vi "Led Control.vi"   [LabVIEW 2013]
uses:
  <vilib>/Rock Robotics/WPI/DriverStation/WPI_DriverStationAllianceInfo.ctl
  <vilib>/Rock Robotics/WPI/Relay/WPI_RelayValue.ctl
types:
  T1 = typedef "WPI_DriverStationAllianceInfo.ctl" = enum16{"Red", "Blue", "Invalid"}
  T2 = typedef "WPI_RelayValue.ctl" = enum16{"Off", "On", "Forward", "Reverse"}
  T3 = typedef "WPI_RelayDevRef.ctl" = cluster{"DevStatus":errorcluster, "Relay Channel":T4, "Digital Module":T5, "Relay Direction":T6}
  T4 = typedef "FPGA_DIORelayChannel.ctl" = enum8{"Relay 1", "Relay 2", "Relay 3", "Relay 4", "Relay 5", "Relay 6", "Relay 7", "Relay 8", "Invalid"}
  T5 = typedef "FPGA_TypedefDigitalModule.ctl" = enum16{"Digital Module 1", "Digital Module 2"}
  T6 = typedef "WPI_RelayDirection.ctl" = enum16{"Both directions", "Forward only", "Reverse only"}
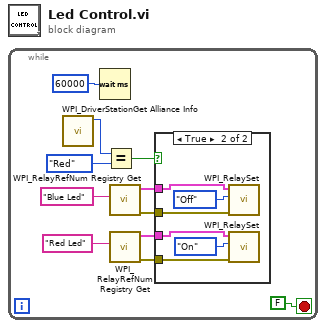
[diagram p0: block diagram]
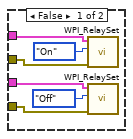
[diagram p2: hidden frame]
diagram:
  n1 = while {
    stop <- FALSE stop-if-true
    n2 = call <vilib>:"WPI_DriverStationGet Alliance Info.vi"() -> ("Alliance"=w6:T1)  [unwired: 10 in, 1 out]
    n3 = Wait (ms)(milliseconds to wait=u32 60000) -> ()  [unwired: 1 out]
    n4 = Equal?(x=w6, y=WPI_DriverStationAllianceInfo."Red" ("Alliance")) -> (x = y?=w7:bool)
    n5 = call <vilib>:"WPI_RelayRefNum Registry Get.vi"("refnum name"="Blue Led") -> ("error out"=w1:errorcluster, "RelayDevRef"=w2:T3)  [unwired: 9 in]
    n6 = call <vilib>:"WPI_RelayRefNum Registry Get.vi"("refnum name"="Red Led") -> ("error out"=w3:errorcluster, "RelayDevRef"=w4:T3)  [unwired: 9 in]
    n7 = case shown="True" w7 {
      tunnel: w4 -> [w13 w23]
      tunnel: w3 -> [w12 w22]
      tunnel: w2 -> [w15 w19]
      tunnel: w1 -> [w14 w18]
      frame False {
        n8 = call <vilib>:"WPI_RelaySet.vi"("error in (no error)"=w14, "RelayValue"=WPI_RelayValue."On", "RelayDevRef"=w15) -> ()  [unwired: 7 in, 2 out]
        n9 = call <vilib>:"WPI_RelaySet.vi"("error in (no error)"=w12, "RelayValue"=WPI_RelayValue."Off", "RelayDevRef"=w13) -> ()  [unwired: 7 in, 2 out]
      }
      frame True {
        n10 = call <vilib>:"WPI_RelaySet.vi"("error in (no error)"=w18, "RelayValue"=WPI_RelayValue."Off", "RelayDevRef"=w19) -> ()  [unwired: 7 in, 2 out]
        n11 = call <vilib>:"WPI_RelaySet.vi"("error in (no error)"=w22, "RelayValue"=WPI_RelayValue."On", "RelayDevRef"=w23) -> ()  [unwired: 7 in, 2 out]
      }
    }
  }
